vi "Auto Align Controller.vi"(10 "Step (in)":i32, 11 "Base Speed":dbl) -> (1 "Step (out)":i32, 2 "Right Speed":dbl, 3 "Left Speed":dbl)   [LabVIEW 2016]
uses:
  Framework/Robot Global Data.vi
  <vilib>/Rock Robotics/Network Tables/NT Read Number.vi
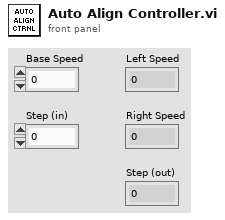
[diagram p1: front panel]
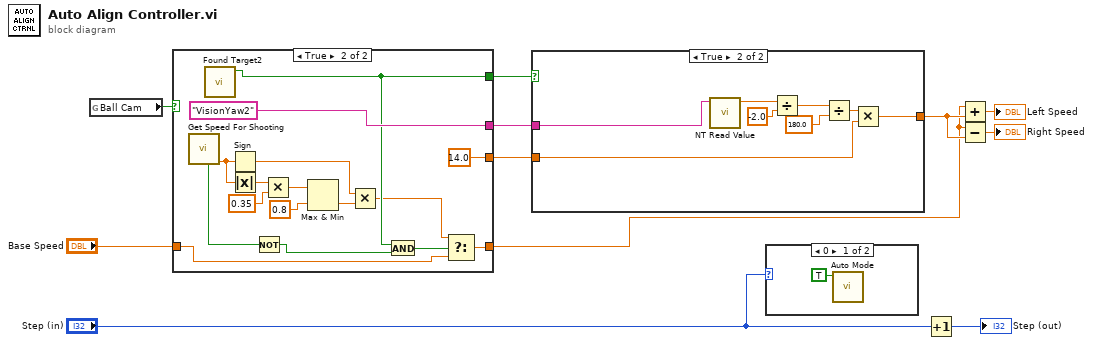
[diagram p0: block diagram]
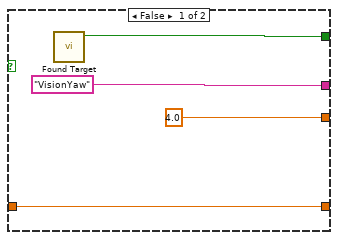
[diagram p3: hidden frame]
diagram:
  n1 = global read "Robot Global Data.vi" "Ball Cam"() -> (w9:bool)
  n2 = case shown="True" w9 {
    tunnel: ["VisionYaw" ("Name") "VisionYaw2" ("Name")] -> w10
    tunnel: [w14 w21] -> w11
    tunnel: "Base Speed" -> [w13 w18]
    tunnel: [w13 w26] -> w1
    tunnel: [4.0 ("y") 14.0 ("y")] -> w3
    frame False {
      n3 = call "Found Target"() -> ("Boolean"=w14:bool)  [unwired: 11 in]
    }
    frame True {
      n4 = call "Get Speed For Shooting.vi"() -> ("Cal Zone Diff"=w27:dbl, "Within Cal Zone?"=w17:bool)  [unwired: 7 in, 3 out]
      n5 = call "Found Target2.vi"() -> ("Boolean"=w21:bool)  [unwired: 11 in]
      n6 = Sign(1:w27) -> (0:w22:dbl)
      n7 = Absolute Value(x=w27) -> (abs(x)=w24:dbl)
      n8 = Not(x=w17) -> (.not. x?=w16:bool)
      n9 = Multiply(x=w24, y=0.35 ("x")) -> (x*y=w28:dbl)
      n10 = Max & Min(x=w28, y=0.8) -> (min(x,y)=w29:dbl)  [unwired: 1 out]
      n11 = Multiply(x=w22, y=w29) -> (x*y=w19:dbl)
      n12 = And(x=w21, y=w16) -> (x .and. y?=w20:bool)
      n13 = Select(t=w19, s=w20, f=w18) -> (s? t:f=w26:dbl)
    }
  }
  n14 = case shown="True" w11 {
    tunnel: [_ w39] -> w2
    tunnel: w10 -> [_ w38]
    tunnel: w3 -> [_ w32]
    frame False {
    }
    frame True {
      n15 = call-poly <vilib>:"NT Read Value.vi"("Name"=w38) -> ("Numeric"=w33:dbl)  [unwired: 9 in, 1 out]
      n16 = Divide(x=w33, y=-2.0) -> (x/y=w35:dbl)
      n17 = Divide(x=w35, y=180.0) -> (x/y=w36:dbl)
      n18 = Multiply(x=w36, y=w32) -> (x*y=w39:dbl)
    }
  }
  n19 = case shown="0" "Step (in)" {
    frame 0 {
      n20 = call "Auto Mode.vi"("Ball?"=TRUE) -> ()  [unwired: 11 in]
    }
    frame 1, Default {
    }
  }
  n21 = Increment(x="Step (in)") -> (x+1=→"Step (out)":i32)
  n22 = Add(x=w1, y=w2) -> (x+y=→"Left Speed":dbl)
  n23 = Subtract(x=w1, y=w2) -> (x-y=→"Right Speed":dbl)
